vi "总磷单步调试对话框.vi"() -> ()   [LabVIEW 2016, in "斯坦道CODcr.lvlib"]
panel:
  in  "停止":bool
  out "注射器温度":sgl
  out "消解温度":sgl
  out "ADC":sgl
  out "F3":sgl format="%#.6f"
  out "F2":sgl format="%#.6f"
  out "F1":sgl format="%#.6f"
  out "F0":sgl format="%#.6f"
  in  "退出":bool
  in  "启动":bool
  in  "总磷氨氮调试":u16[](xcontrol)
  # "单步调试界面"
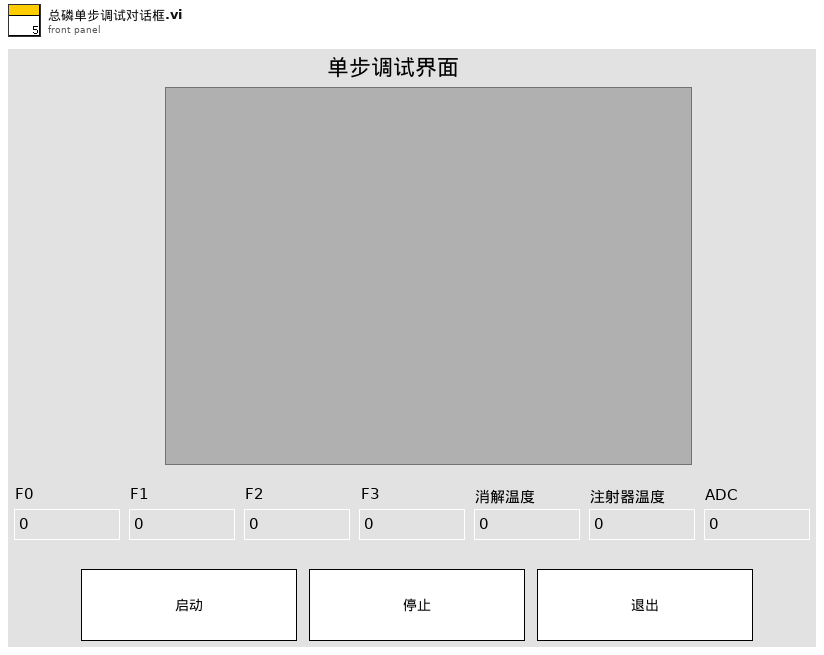
[diagram p1: front panel]
types:
  T1 = cluster{"阀口名称自定义类型":enum16{"自定义", "微站总磷总氮", "微站总磷氨氮", "微站氨氮", "固定站总磷", "固定站总氮", "固定站氨氮", "原位总磷总氮", "原位总磷氨氮", "原位总磷", "原位总氮", "原位氨氮", "原位3N1P"}, "阀口自定义名称":cluster{"V1":string, "V2":string, "V3":string, "V4":string, "V5":string, "V6":string, "V7":string, "V8":string, "V9":string, "V10":string, "V11":string, "V12":string, "V9-1":string, "V9-2":string, "COD慢速":string}}
  T2 = enum16{"自定义", "微站总磷总氮", "微站总磷氨氮", "微站氨氮", "固定站总磷", "固定站总氮", "固定站氨氮", "原位总磷总氮", "原位总磷氨氮", "原位总磷", "原位总氮", "原位氨氮", "原位3N1P"}
  T3 = cluster{"V1":string, "V2":string, "V3":string, "V4":string, "V5":string, "V6":string, "V7":string, "V8":string, "V9":string, "V10":string, "V11":string, "V12":string, "V9-1":string, "V9-2":string, "COD慢速":string}
  T4 = cluster{"系统时间":timestamp, "工作状态":u16, "测量模式":enum16{"待机", "连续模式", "周期模式", "定点模式", "受控模式", "手动模式"}, "告警代码":u16, "故障代码":u16, "日志代码":u16, "软件版本":u16, "F0":sgl, "F1":sgl, "F2":sgl, "F3":sgl, "T":sgl, "H":sgl, "id":u16, "flowid":u16, "量程":u16, "总磷控温温度1":sgl, "营养盐控温温度2":sgl, "ADC":sgl}
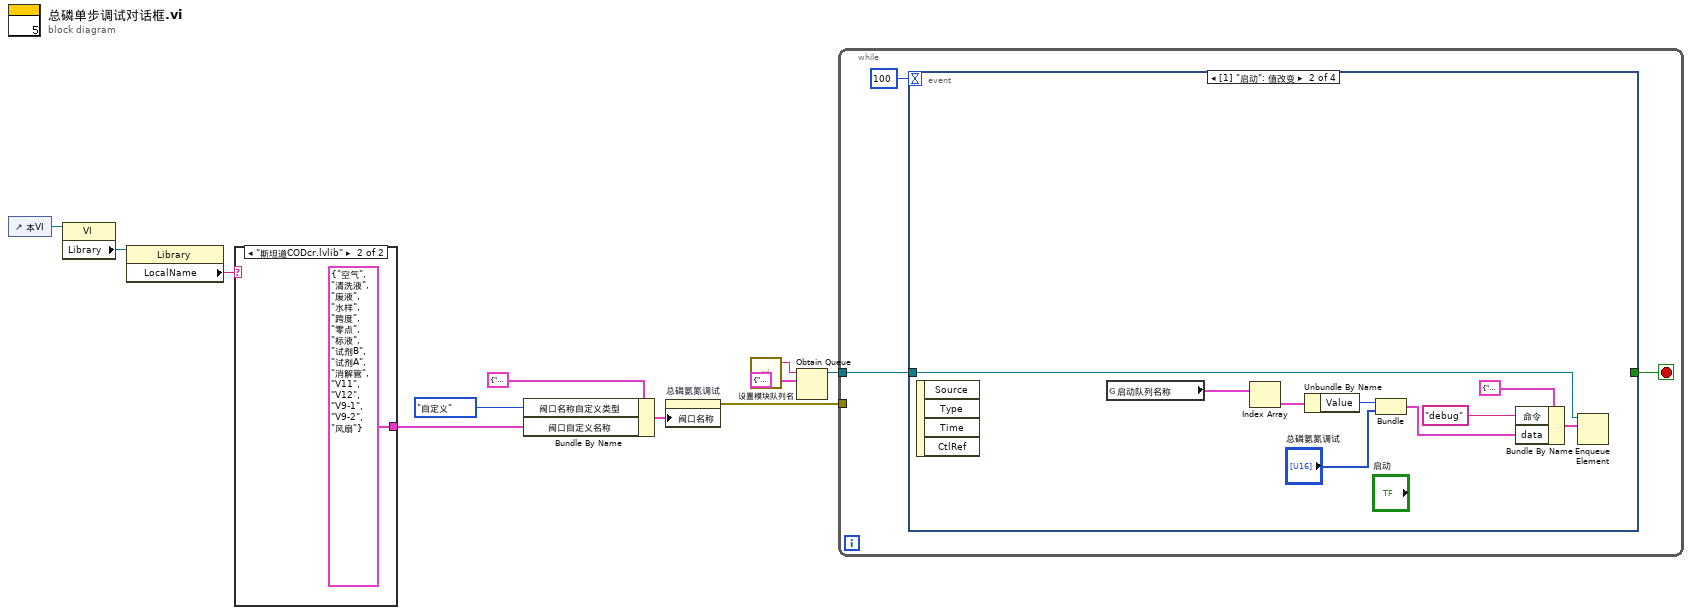
[diagram p0: block diagram]
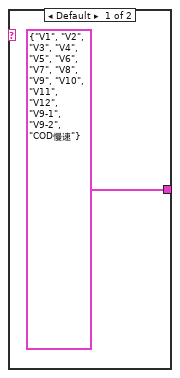
[diagram p2: hidden frame]
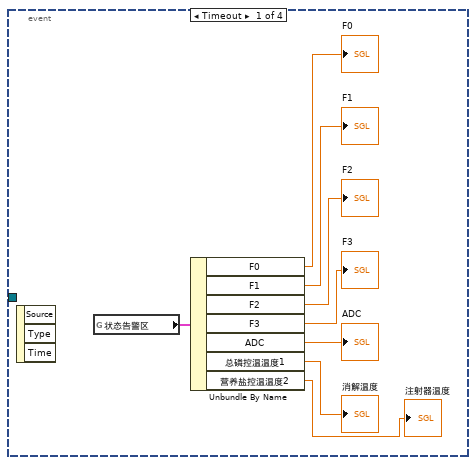
[diagram p3: hidden frame]
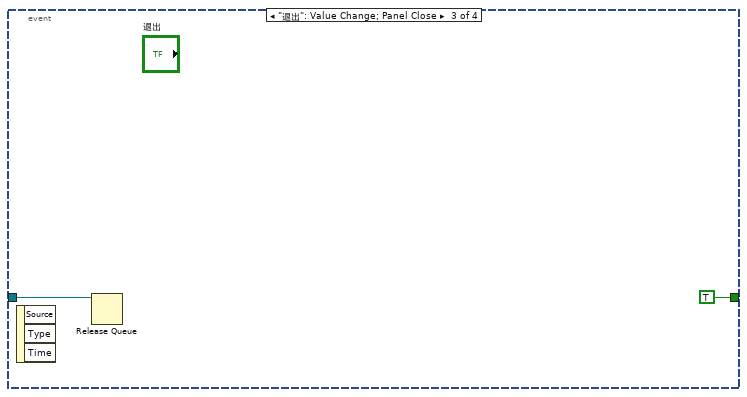
[diagram p4: hidden frame]
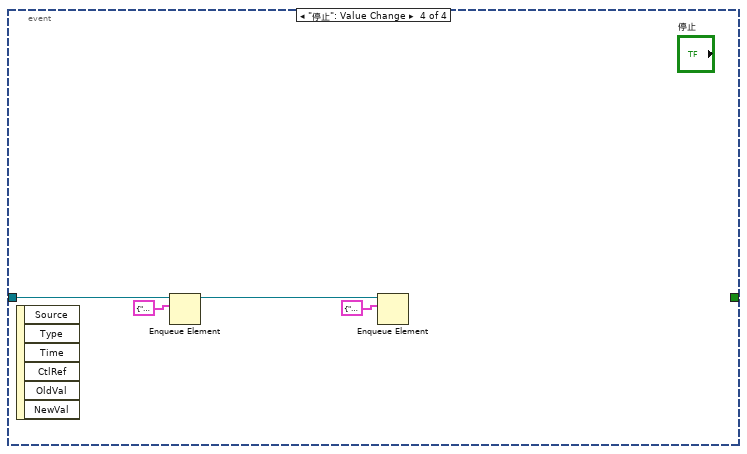
[diagram p5: hidden frame]
diagram:
  n1 = control-ref of="本VI"() -> (w5:refnum<vi>)
  n2 = property class="VI"(reference=w5) -> ("Library"=w6:refnum<vi>)  [unwired: 1 in, 2 out]
  n3 = property class="Library"(reference=w6) -> ("LocalName"=w4:string)  [unwired: 1 in, 2 out]
  n4 = case shown="\"斯坦道CODcr.lvlib\"" w4 {
    tunnel: [T3 {"V1"="V1", "V2"="V2", "V3"="V3", "V4"="V4", "V5"="V5", "V6"="V6", "V7"="V7", "V8"="V8", "V9"="V9", "V10"="V10", "V11"="V11", "V12"="V12", "V9-1"="V9-1", "V9-2"="V9-2", "COD慢速"="COD慢速"} ("阀口自定义名称") T3 {"V1"="空气", "V2"="清洗液", "V3"="废液", "V4"="水样", "V5"="跨度", "V6"="零点", "V7"="标液", "V8"="试剂B", "V9"="试剂A", "V10"="消解管", "V11"="V11", "V12"="V12", "V9-1"="V9-1", "V9-2"="V9-2", "COD慢速"="风扇"} ("阀口自定义名称")] -> w1
    frame Default {
    }
    frame "斯坦道CODcr.lvlib" {
    }
  }
  n5 = Bundle By Name(cluster=T1 {"阀口名称自定义类型"=enum."自定义", "阀口自定义名称"={"V1"="", "V2"="", "V3"="", "V4"="", "V5"="", "V6"="", "V7"="", "V8"="", "V9"="", "V10"="", "V11"="", "V12"="", "V9-1"="", "V9-2"="", "COD慢速"=""}} ("阀口名称"), "阀口名称自定义类型"=T2."自定义", "阀口自定义名称"=w1) -> (w3:T1)
  n6 = property on="总磷氨氮调试" class="调试控件V3 (严格)"("阀口名称"=w3) -> (error out=w9:errorcluster)  [unwired: 2 in, 1 out]
  n7 = call "设置模块队列名.vi"() -> ("Msg"=w7:string)  [unwired: 5 in]
  n8 = Obtain Queue(name (unnamed)=w7, element data type=cluster{"命令":string, "data":variant} {"命令"="", "data"=variant}) -> (queue out=w10:refnum<queue>)  [unwired: 3 in, 2 out]
  n9 = while {
    tunnel: w10 -> [w16]
    tunnel: w9 -> [_]
    stop <- w15 stop-if-true
    n10 = event shown="[1] \"启动\": 值改变" {
      selector: _ -> [_ _ _ _]
      dyn-events: _ -> [_ _ _ _]
      timeout: 100 -> [_ _ _ _]
      tunnel: w16 -> [_ w29 w34 w36]
      tunnel: [_ _ TRUE _] -> w15
      event Timeout {
        n11 = event-data() -> ()  [unwired: 1 in, 3 out]
        n12 = global read "VAR总磷总氮全局变量.vi" "状态告警区"() -> (w17:T4)
        n13 = Unbundle By Name(w17) -> ("F0"=→"F0":sgl, "F1"=→"F1":sgl, "F2"=→"F2":sgl, "F3"=→"F3":sgl, "ADC"=→"ADC":sgl, "总磷控温温度1"=→"消解温度":sgl, "营养盐控温温度2"=→"注射器温度":sgl)
      }
      event "启动": Value Change {
        n14 = event-data() -> ()  [unwired: 1 in, 4 out]
        n15 = global read "总磷总氮断电保存全局变量.vi" "启动队列名称"() -> (w25:cluster{"String":string, "Value":u16}[])
        n16 = Index Array(array=w25) -> (element=w27:cluster{"String":string, "Value":u16})  [unwired: 1 in]
        n17 = Unbundle By Name(w27) -> ("Value"=w26:u16)
        n18 = Bundle("Value"=w26, "总磷氨氮调试"="总磷氨氮调试") -> (w30:cluster{"Value":u16, "总磷氨氮调试":u16[]})  [unwired: 1 in]
        n19 = Bundle By Name(cluster=cluster{"命令":string, "data":variant} {"命令"="", "data"=variant} ("元素"), "命令"="debug", "data"=w30) -> (w31:cluster{"命令":string, "data":variant})
        n20 = Enqueue Element(queue=w29, element=w31) -> ()  [unwired: 2 in, 3 out]
      }
      event "退出": Value Change; Panel Close {
        n21 = event-data() -> ()  [unwired: 1 in, 3 out]
        n22 = Release Queue(queue=w34) -> ()  [unwired: 2 in, 3 out]
      }
      event "停止": Value Change {
        n23 = event-data() -> ()  [unwired: 1 in, 6 out]
        n24 = Enqueue Element(queue=w36, element=cluster{"命令":string, "data":variant} {"命令"="启动", "data"=variant(cluster{"站号":u16, "控制命令输出":u16[]} {"站号"=1, "控制命令输出"=[2816]})} ("元素")) -> (queue out=w37:refnum<queue>)  [unwired: 2 in, 2 out]
        n25 = Enqueue Element(queue=w37, element=cluster{"命令":string, "data":variant} {"命令"="启动", "data"=variant(cluster{"站号":u16, "控制命令输出":u16[]} {"站号"=2, "控制命令输出"=[2816]})} ("元素")) -> ()  [unwired: 2 in, 3 out]
      }
    }
  }
